vi "matrici_v0_v20.vi"() -> ()   [LabVIEW 2009]
panel:
  out "Numeric":dbl
  in  "stop":bool
  out "Picture":picture
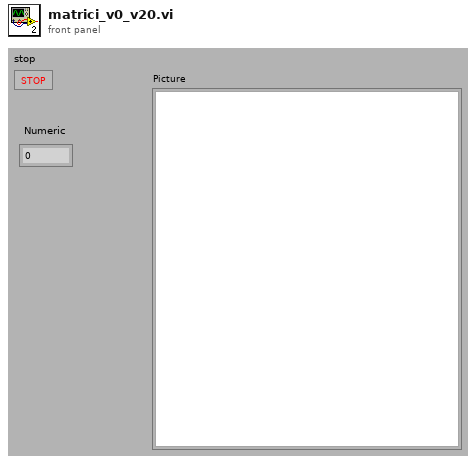
[diagram p1: front panel]
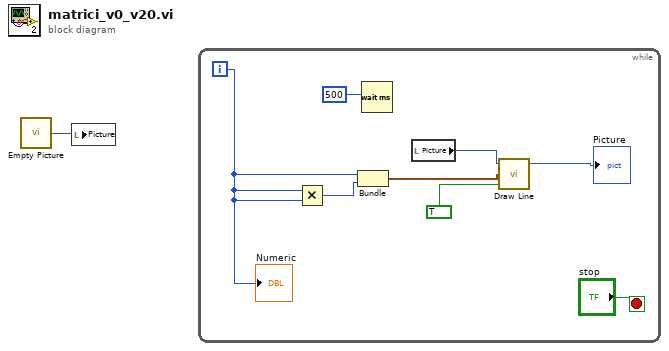
[diagram p0: block diagram]
diagram:
  n1 = call "Empty Picture"() -> ("empty picture"=w1:picture)
  n2 = local write "Picture"(w1) -> ()
  n3 = while {
    i -> [w2]
    stop <- "stop" stop-if-true
    n4 = Multiply(x=w2, y=w2) -> (x*y=w3:i32)
    n5 = Bundle(w2, w3) -> (w6:cluster{i32, i32})  [unwired: 1 in]
    n6 = Wait (ms)(milliseconds to wait=500) -> ()  [unwired: 1 out]
    n7 = local read "Picture"() -> (w8:picture)
    n8 = call <vilib>:"Draw Line.vi"("picture"=w8, "end point"=w6, "absolute coordinates?(T)"=TRUE) -> ("new picture"=→"Picture":picture)  [unwired: 6 in]
    "Numeric" <- w2
  }
